vi "SendTCPString.vi"(8 "error in (no error)":errorcluster, 10 "String":string, 11 "TCP Network Connection in":refnum<k5>) -> (0 "error out":errorcluster)   [LabVIEW 2019]
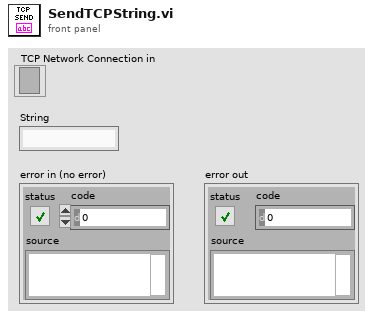
[diagram p1: front panel]
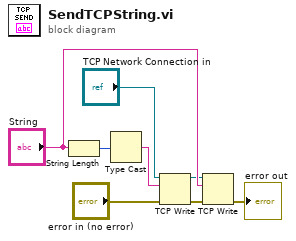
[diagram p0: block diagram]
diagram:
  n1 = String Length(string="String") -> (length=w1:i32)
  n2 = Type Cast(x=w1) -> (*(type *) &x=w3:string)  [unwired: 1 in]
  n3 = TCP Write(connection ID="TCP Network Connection in", data in=w3, error in (no error)="error in (no error)") -> (connection ID out=w5:refnum<k5>, error out=w4:errorcluster)  [unwired: 1 in, 1 out]
  n4 = TCP Write(connection ID=w5, data in="String", error in (no error)=w4) -> (error out=→"error out":errorcluster)  [unwired: 1 in, 2 out]
